vi "SECoP_dataCreate.vi"(8 "error in (no error)":errorcluster, 10 "Description":string, 11 "DLL path (in)":T2) -> (0 "error out":errorcluster, 2 "SECoP_dataPtr (out)":T1 {"ptr64" format="%.0x"; "ptr32" format="%.0x"}, 3 "DLL path (out)":T2)   [LabVIEW 2023, in "SECoP.lvlib"]
doc: "Call <b>\"SECoP_dataCreate.vi\"</b> to create a new value with the described data type. See SECoP protocol definition. Free resources after use with <b>\"SECoP_dataDestroy.vi\"</b>.\n\n<b>DLL path</b> input and output of cluster from \"SECoP-Initialize.vi\"\n<b>Description</b> SECoP data type description\n<b>SECoP_dataPtr</b> created data"
uses:
  SECoP.lvlib
  SECoP-libraries.ctl
  SECoP-data.ctl
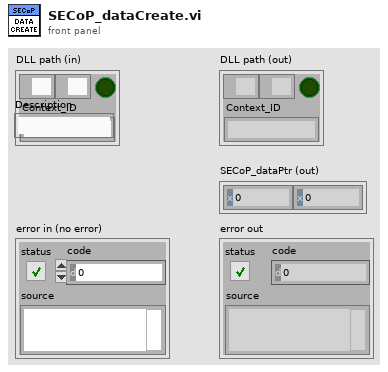
[diagram p1: front panel]
types:
  T1 = typedef "SECoP.lvlib/SECoP-data.ctl" = cluster{"ptr32":u32, "ptr64":u64}
  T2 = typedef "SECoP.lvlib/SECoP-libraries.ctl" = cluster{"serverDLL":path, "variantDLL":path, "cleanup_mode":bool, "Context_ID":string}
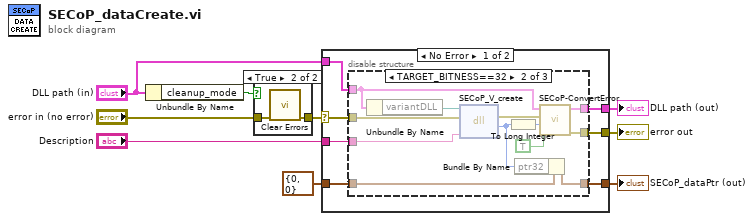
[diagram p0: block diagram]
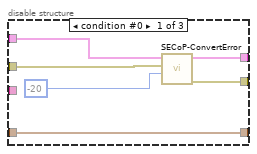
[diagram p3: hidden frame]
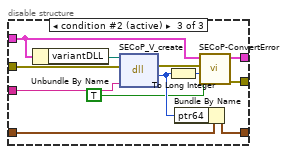
[diagram p4: hidden frame]
diagram:
  n1 = Unbundle By Name("DLL path (in)") -> ("cleanup_mode"=w7:bool)
  n2 = case shown="True" w7 {
    tunnel: "error in (no error)" -> [w10 w12]
    tunnel: [w10 w11] -> w5
    frame False {
    }
    frame True {
      n3 = call <vilib>:"Clear Errors.vi"("error in (no error)"=w12) -> ("error out"=w11:errorcluster)  [unwired: 5 in, 1 out]
    }
  }
  n4 = case shown="No Error" w5 {
    selector: w5 -> [w19 w51]
    tunnel: "DLL path (in)" -> [w18 w52]
    tunnel: [w16 w52] -> w9
    tunnel: [w17 w51] -> w8
    tunnel: "Description" -> [w15 _]
    tunnel: [w13 w50] -> w3
    tunnel: T1 {"ptr32"=0, "ptr64"=0} ("SECoP_dataPtr (out)") -> [w14 w50]
    frame No Error {
      n5 = disable-structure shown="TARGET_BITNESS==32" {
        disable-tunnel: w19 -> [w25 w37 w49]
        disable-tunnel: w18 -> [w24 w26 w38]
        disable-tunnel: [w22 w32 w44] -> w17
        disable-tunnel: [w23 w31 w43] -> w16
        disable-tunnel: w15 -> [_ w36 w48]
        disable-tunnel: w14 -> [w20 w34 w46]
        disable-tunnel: [w20 w35 w47] -> w13
        frame condition #0 {
          n6 = call "SECoP-ConvertError.vi"("return code"=-20, "error in (no error)"=w25, "DLL path (in)"=w24) -> ("error out"=w22:errorcluster, "DLL path (out)"=w23:T2)  [unwired: 7 in]
        }
        frame condition #1 {
          n7 = Unbundle By Name(w26) -> ("variantDLL"=w27:path)
          n8 = dll-call lib="Z:/Praktische_Aufgaben/SECoP-LabVIEW2015/32bit/SECoP32.dll" fn="SECoP_V_create"(path in=w27, error in=w37, "Description"=w36) -> (error out=w33:errorcluster, "return type"=w30:u32)  [unwired: 2 in, 1 out]
          n9 = To Long Integer(number=w30) -> (32bit integer=w28:i32)
          n10 = Bundle By Name(cluster=w34, "ptr32"=w30) -> (w35:T1)
          n11 = call "SECoP-ConvertError.vi"("return is boolean"=TRUE, "return code"=w28, "error in (no error)"=w33, "DLL path (in)"=w26) -> ("error out"=w32:errorcluster, "DLL path (out)"=w31:T2)  [unwired: 6 in]
        }
        frame condition #2 (active) {
          n12 = Unbundle By Name(w38) -> ("variantDLL"=w39:path)
          n13 = dll-call lib="Z:/Praktische_Aufgaben/SECoP-LabVIEW2015/32bit/SECoP32.dll" fn="SECoP_V_create"(path in=w39, error in=w49, "Description"=w48) -> (error out=w45:errorcluster, "return type"=w42:u64)  [unwired: 2 in, 1 out]
          n14 = To Long Integer(number=w42) -> (32bit integer=w40:i32)
          n15 = Bundle By Name(cluster=w46, "ptr64"=w42) -> (w47:T1)
          n16 = call "SECoP-ConvertError.vi"("return is boolean"=TRUE, "return code"=w40, "error in (no error)"=w45, "DLL path (in)"=w38) -> ("error out"=w44:errorcluster, "DLL path (out)"=w43:T2)  [unwired: 6 in]
        }
      }
    }
    frame Error {
    }
  }
  "DLL path (out)" <- w9
  "error out" <- w8
  "SECoP_dataPtr (out)" <- w3
